vi "Line separate.vi"(10 "Y array":dbl[](array[numeric]), 11 "X array":dbl[](array[numeric])) -> (0 "Global Line Map":cluster{dbl[], dbl[]}[](graph), 2 "Line Seg Array":dbl[][][](array[numeric]), 3 "Wall Seg Array":dbl[][][](array[numeric]))   [LabVIEW 2018]
panel:
  in  "Length Diff Ratio":dbl=1.5
  in  "Slope Diff Ratio":dbl=0.5
  out "x-1":i32
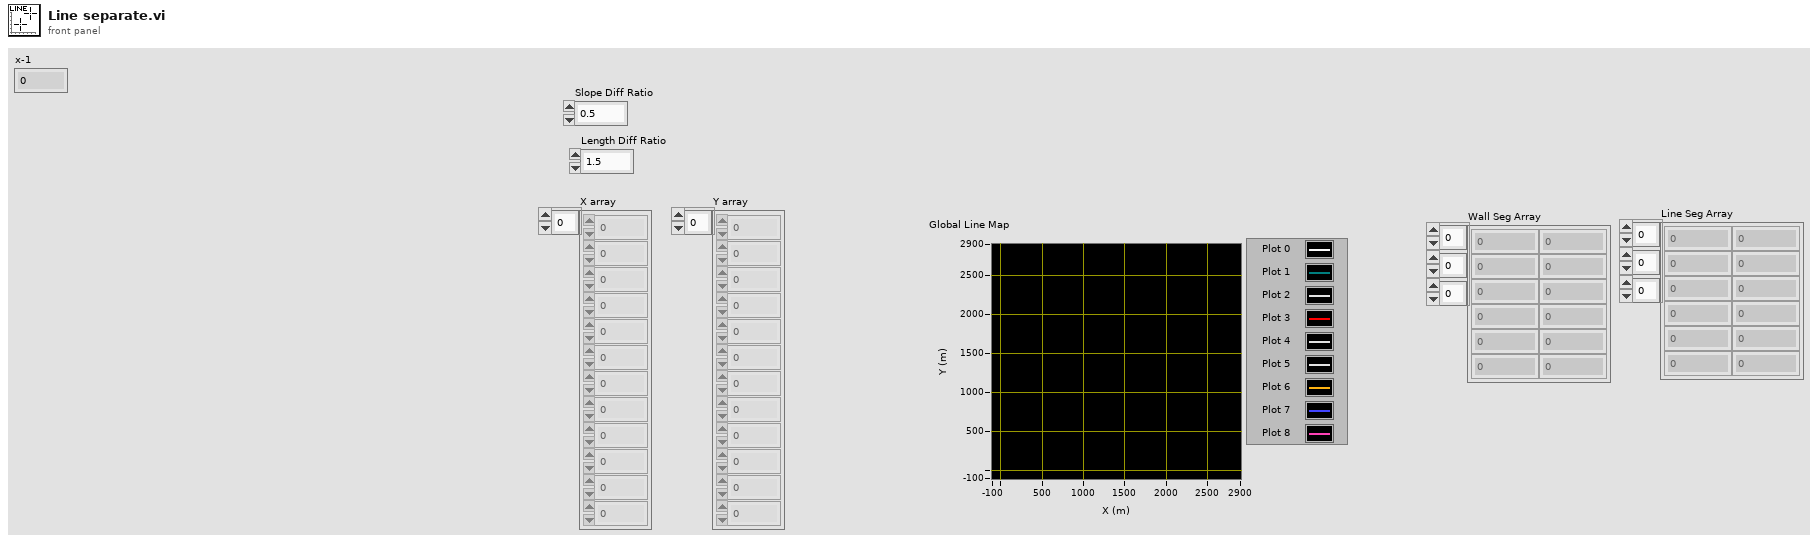
[diagram p1: front panel]
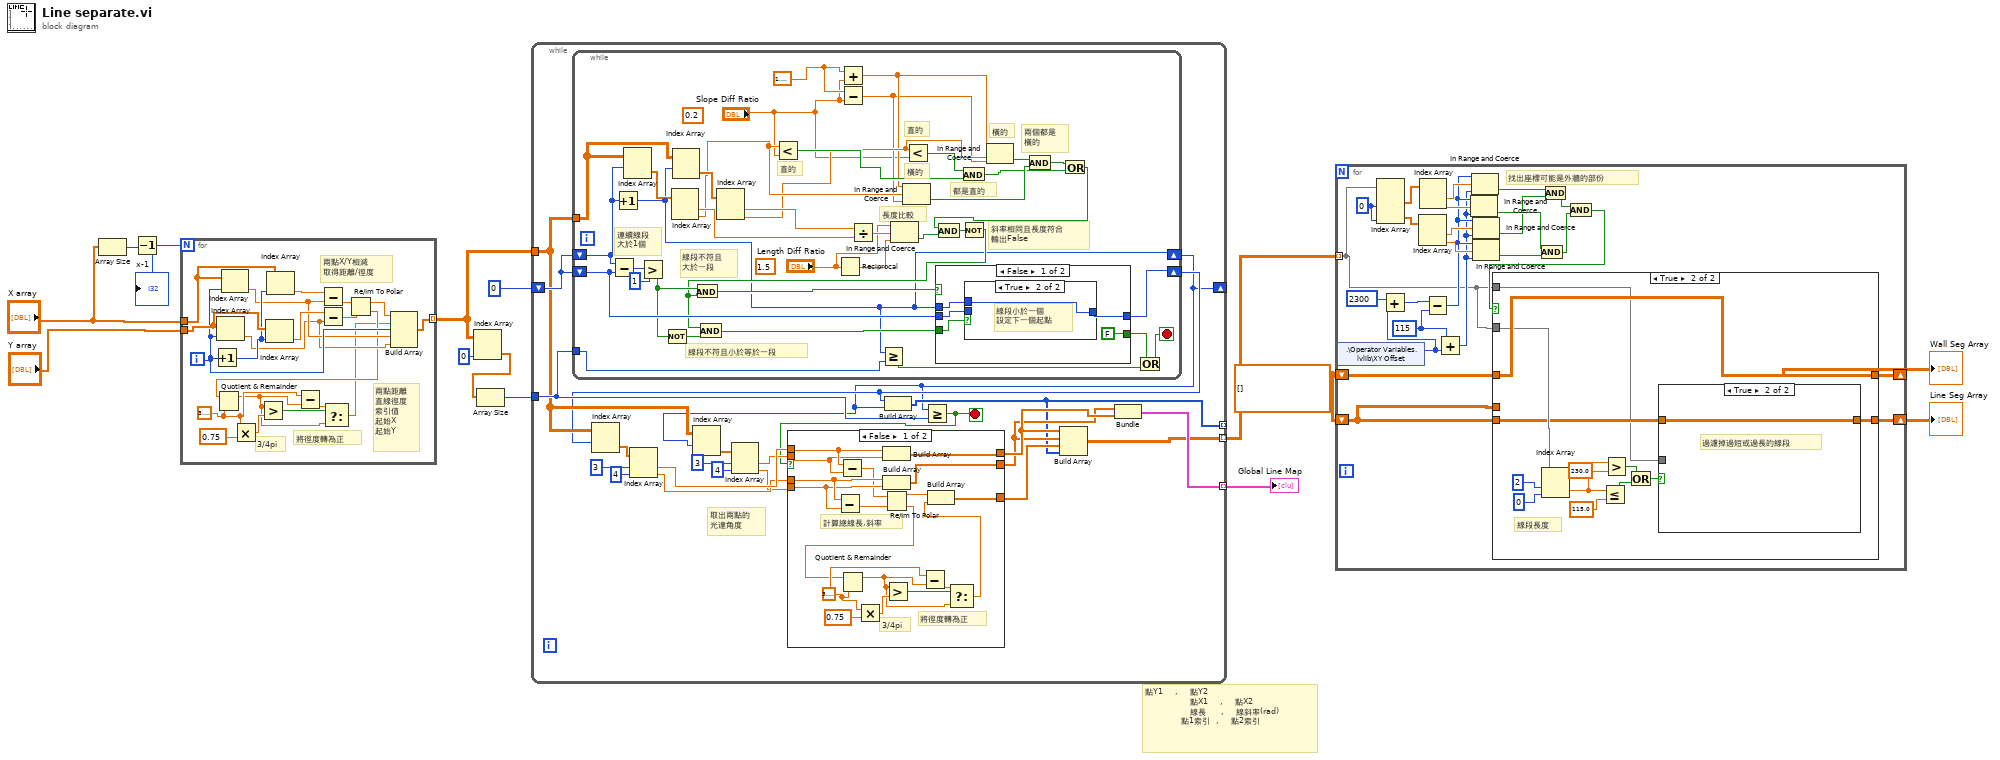
[diagram p0: block diagram]
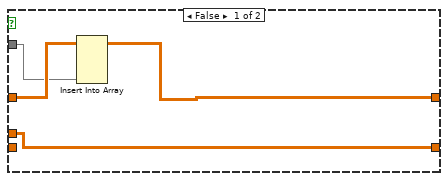
[diagram p2: hidden frame]
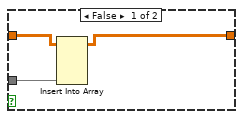
[diagram p3: hidden frame]
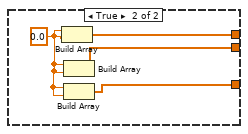
[diagram p4: hidden frame]
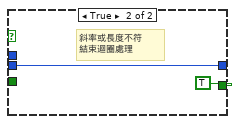
[diagram p6: hidden frame]
diagram:
  w5 = dbl[][][] [] ("Array 6")
  # "點Y1    ,    點Y2    \n               點X1    ,    點X2\n               線長     ,    線斜率(rad)\n            點1索引  ,    點2索引"
  n1 = Array Size(array="X array") -> (size(s)=w14:i32)
  n2 = Decrement(x=w14) -> (x-1=w13:i32)
  "x-1" <- w13
  n3 = for {
    N: w13 -> [_]
    tunnel: [w33] -> w1 mode=indexing
    tunnel: "X array" -> [w30]
    tunnel: "Y array" -> [w29]
    i -> [w27]
    w17 = 3.141592653589793
    # "將徑度轉為正"
    # "兩點X/Y相減\n取得距離/徑度"
    # "兩點距離\n直線徑度\n索引值\n起始X\n起始Y"
    # "3/4pi"
    n4 = Increment(x=w27) -> (x+1=w28:i32)
    n5 = Index Array(array=w29, index=w27) -> (element=w23:dbl)
    n6 = Index Array(array=w30, index=w27) -> (element=w24:dbl)
    n7 = Multiply(x=w17, y=0.75) -> (x*y=w19:dbl)
    n8 = Index Array(array=w29, index=w28) -> (element=w25:dbl)
    n9 = Index Array(array=w30, index=w28) -> (element=w26:dbl)
    n10 = Subtract(x=w26, y=w24) -> (x-y=w32:dbl)
    n11 = Subtract(x=w25, y=w23) -> (x-y=w31:dbl)
    n12 = Re/Im To Polar(2:w31, 3:w32) -> (0:w22:dbl, 1:w34:dbl)
    n13 = Quotient & Remainder(x=w22, y=w17) -> (x-y*floor(x/y)=w16:dbl)  [unwired: 1 out]
    n14 = Greater?(x=w16, y=w19) -> (0:w20:bool)
    n15 = Subtract(x=w17, y=w16) -> (x-y=w18:dbl)
    n16 = Select(t=w18, s=w20, f=w16) -> (s? t:f=w15:dbl)
    n17 = Build Array(w34, w15, w27, w24, w23) -> (w33:dbl[])
  }
  n18 = Index Array(array=w1, index (col)=0 ("disabled index (col)")) -> (element=w10:dbl[])  [unwired: 1 in]
  n19 = Array Size(array=w10) -> (size(s)=w11:i32)
  n20 = while {
    shift-right: [w35] -> _
    shift-left: 0 -> [w56]
    tunnel: w1 -> [w54]
    tunnel: w11 -> [w55]
    tunnel: [w37] -> _ mode=indexing
    tunnel: [w43] -> w8 mode=indexing
    tunnel: [w39] -> w7 mode=indexing
    stop <- w42 stop-if-true
    # "取出兩點的\n光達角度"
    n21 = while {
      shift-right: [w79] -> w35
      shift-left: w56 -> [w99]
      tunnel: w54 -> [w116]
      tunnel: w55 -> [w96]
      shift-right: [w107] -> w36
      shift-left: w56 -> [w108]
      stop <- w101 stop-if-true
      w86 = 1.5707963267948966
      (unwired) 0.2 ("y")
      (unwired) 1.5 ("upper limit")
      # "線段不符且\n大於一段"
      # "線段不符且小於等於一段"
      # "斜率相同且長度符合\n輸出False"
      # "連續線段\n大於1個"
      # "都是直的"
      # "長度比較"
      # "橫的"
      # "直的"
      # "橫的"
      # "直的"
      # "兩個都是\n橫的"
      n22 = Subtract(x=w99, y=w108) -> (x-y=w110:i32)
      n23 = Increment(x=w99) -> (x+1=w79:i32)
      n24 = Index Array(array=w116, index (row)=w99) -> (element=w115:dbl[])  [unwired: 1 in]
      n25 = Greater?(x=w110, y=1) -> (0:w104:bool)
      n26 = Not(x=w104) -> (.not. x?=w105:bool)
      n27 = Index Array(array=w115) -> (element #1=w112:dbl, element #2=w88:dbl)  [unwired: 2 in]
      n28 = Index Array(array=w116, index (row)=w79) -> (element=w114:dbl[])  [unwired: 1 in]
      n29 = Index Array(array=w114) -> (element #1=w113:dbl, element #2=w87:dbl)  [unwired: 2 in]
      n30 = Less?(x=w88, y="Slope Diff Ratio") -> (x < y?=w92:bool)
      n31 = Reciprocal(x="Length Diff Ratio") -> (1/x=w81:dbl)
      n32 = Add(x=w86, y="Slope Diff Ratio") -> (x+y=w85:dbl)
      n33 = Subtract(x=w86, y="Slope Diff Ratio") -> (x-y=w84:dbl)
      n34 = Divide(x=w113, y=w112) -> (x/y=w111:dbl)
      n35 = Greater Or Equal?(x=w79, y=w96) -> (x >= y?=w100:bool)
      n36 = In Range and Coerce(upper limit="Length Diff Ratio", x=w111, lower limit=w81) -> (In Range?=w98:bool)  [unwired: 1 out]
      n37 = In Range and Coerce(upper limit=w85, x=w88, lower limit=w84) -> (In Range?=w94:bool)  [unwired: 1 out]
      n38 = Less?(x=w87, y="Slope Diff Ratio") -> (x < y?=w93:bool)
      n39 = And(x=w93, y=w92) -> (x .and. y?=w91:bool)
      n40 = In Range and Coerce(upper limit=w85, x=w87, lower limit=w84) -> (In Range?=w95:bool)  [unwired: 1 out]
      n41 = And(x=w95, y=w94) -> (x .and. y?=w89:bool)
      n42 = Or(x=w89, y=w91) -> (x .or. y?=w90:bool)
      n43 = And(x=w90, y=w98) -> (x .and. y?=w97:bool)
      n44 = Not(x=w97) -> (.not. x?=w82:bool)
      n45 = And(x=w104, y=w82) -> (x .and. y?=w106:bool)
      n46 = And(x=w82, y=w105) -> (x .and. y?=w103:bool)
      n47 = case shown="False" w106 {
        tunnel: [FALSE TRUE] -> w102
        tunnel: w108 -> [w119 w124]
        tunnel: w79 -> [w118 _]
        tunnel: [w117 w124] -> w107
        tunnel: w103 -> [w120 _]
        frame False {
          n48 = case shown="True" w120 {
            tunnel: w119 -> [w122 _]
            tunnel: w118 -> [_ w123]
            tunnel: [w122 w123] -> w117
            frame False {
              # "線段符合,繼續處理\n維持起始點"
            }
            frame True {
              # "線段小於一個\n設定下一個起點"
            }
          }
        }
        frame True {
          # "斜率或長度不符\n結束迴圈處理"
        }
      }
      n49 = Or(x=w102, y=w100) -> (x .or. y?=w101:bool)
    }
    n50 = Index Array(array=w54, index (row)=w36) -> (element=w53:dbl[])  [unwired: 1 in]
    n51 = Index Array(array=w53, index #1=3 ("index"), index #2=4 ("index")) -> (element #1=w47:dbl, element #2=w45:dbl)
    n52 = Index Array(array=w54, index (row)=w35) -> (element=w48:dbl[])  [unwired: 1 in]
    n53 = Index Array(array=w48, index #1=3 ("index"), index #2=4 ("index")) -> (element #1=w46:dbl, element #2=w44:dbl)
    n54 = Build Array(w36, w35) -> (w37:i32[])
    n55 = Greater Or Equal?(x=w35, y=w55) -> (x >= y?=w42:bool)
    n56 = case shown="False" w42 {
      tunnel: w47 -> [w72 _]
      tunnel: w46 -> [w71 _]
      tunnel: w45 -> [w70 _]
      tunnel: w44 -> [w69 _]
      tunnel: [w74 w78] -> w41
      tunnel: [w73 w77] -> w40
      tunnel: [w65 w75] -> w38
      frame False {
        w60 = 3.141592653589793
        # "將徑度轉為正"
        # "3/4pi"
        # "計算總線長,斜率"
        n57 = Subtract(x=w70, y=w69) -> (x-y=w67:dbl)
        n58 = Subtract(x=w72, y=w71) -> (x-y=w68:dbl)
        n59 = Multiply(x=w60, y=0.75) -> (x*y=w63:dbl)
        n60 = Build Array(w72, w71) -> (w74:dbl[])
        n61 = Build Array(w70, w69) -> (w73:dbl[])
        n62 = Re/Im To Polar(2:w67, 3:w68) -> (0:w58:dbl, 1:w66:dbl)
        n63 = Quotient & Remainder(x=w58, y=w60) -> (x-y*floor(x/y)=w61:dbl)  [unwired: 1 out]
        n64 = Greater?(x=w61, y=w63) -> (0:w64:bool)
        n65 = Subtract(x=w60, y=w61) -> (x-y=w62:dbl)
        n66 = Select(t=w62, s=w64, f=w61) -> (s? t:f=w57:dbl)
        n67 = Build Array(w66, w57) -> (w65:dbl[])
      }
      frame True {
        w76 = 0.0
        n68 = Build Array(w76, w76) -> (w78:dbl[])
        n69 = Build Array(w76, w76) -> (w77:dbl[])
        n70 = Build Array(w76, w76) -> (w75:dbl[])
      }
    }
    n71 = Build Array(w41, w40, w38, w37) -> (w39:dbl[][])
    n72 = Bundle(w40, w41) -> (w43:cluster{dbl[], dbl[]})  [unwired: 1 in]
  }
  "Global Line Map" <- w8
  n73 = for {
    tunnel: w7 -> [w126] mode=indexing
    shift-right: [w135] -> w2
    shift-left: w5 -> [w137]
    shift-right: [w136] -> w6
    shift-left: w5 -> [w127]
    w144 = i16 115 ("x")
    w149 = 0 ("disabled index (row)")
    # "找出座標可能是外牆的部份"
    n74 = shared-variable ".\\Operator Variables.lvlib\\XY Offset"() -> (w146:i16)  [unwired: 1 in, 1 out]
    n75 = Index Array(array=w126, index (col) #1=w149, index (col) #2=w149) -> (element #1=w150:dbl[], element #2=w148:dbl[])  [unwired: 2 in]
    n76 = Add(x=i16 2300, y=w146) -> (x+y=w145:i16)
    n77 = Index Array(array=w148) -> (element #1=w141:dbl, element #2=w140:dbl)  [unwired: 2 in]
    n78 = Index Array(array=w150) -> (element #1=w143:dbl, element #2=w142:dbl)  [unwired: 2 in]
    n79 = Subtract(x=w145, y=w144) -> (x-y=w139:i16)
    n80 = Add(x=w144, y=w146) -> (x+y=w138:i16)
    n81 = In Range and Coerce(upper limit=w139, x=w142, lower limit=w138) -> (In Range?=w134:bool)  [unwired: 1 out]
    n82 = In Range and Coerce(upper limit=w139, x=w143, lower limit=w138) -> (In Range?=w132:bool)  [unwired: 1 out]
    n83 = In Range and Coerce(upper limit=w139, x=w141, lower limit=w138) -> (In Range?=w131:bool)  [unwired: 1 out]
    n84 = In Range and Coerce(upper limit=w139, x=w140, lower limit=w138) -> (In Range?=w133:bool)  [unwired: 1 out]
    n85 = And(x=w134, y=w133) -> (x .and. y?=w129:bool)
    n86 = And(x=w132, y=w131) -> (x .and. y?=w130:bool)
    n87 = And(x=w130, y=w129) -> (x .and. y?=w128:bool)
    n88 = case shown="True" w128 {
      tunnel: w126 -> [w151 w166]
      tunnel: w137 -> [w152 w167]
      tunnel: w127 -> [w153 _]
      tunnel: [w154 w167] -> w135
      tunnel: [w153 w155] -> w136
      tunnel: w127 -> [_ w157]
      tunnel: w126 -> [_ w156]
      frame False {
        n89 = Insert Into Array(array=w152, new element=w151) -> (w154:dbl[][][])  [unwired: 3 in]
      }
      frame True {
        # "線段長度"
        n90 = Index Array(array=w166, index (row)=2, index (col)=0 ("disabled index (col)")) -> (element=w162:dbl)
        n91 = Less Or Equal?(x=w162, y=115.0) -> (x <= y?=w159:bool)
        n92 = Greater?(x=w162, y=230.0) -> (0:w160:bool)
        n93 = Or(x=w160, y=w159) -> (x .or. y?=w158:bool)
        n94 = case shown="True" w158 {
          tunnel: w157 -> [w170 w171]
          tunnel: w156 -> [w169 _]
          tunnel: [w168 w171] -> w155
          frame False {
            n95 = Insert Into Array(array=w170, new element=w169) -> (w168:dbl[][][])  [unwired: 3 in]
          }
          frame True {
            # "過濾掉過短或過長的線段"
          }
        }
      }
    }
  }
  "Line Seg Array" <- w6
  "Wall Seg Array" <- w2
